vi "InitializeMaskLoad.vi"(4 "dxfFile":string, 5 "Masks":string, 6 "WaferTestPoints":string, 7 "DXFCanvas":refnum<k24>, 9 "TestPointsLoaded":bool, 10 "Wafer Definition File":path, 11 "MicrositesRef":refnum<k24>) -> (0 "error out":errorcluster, 3 "error out 5":errorcluster)   [LabVIEW 2020]
uses:
  C:/Users/User/Desktop/Automation/NextVersion/DXFViewer/LabviewDXFViewer/LabviewDXFViewer/bin/Release/LabviewDXFViewer.exe
  LabviewDXFViewer/bin/Release/LabviewDXFViewer.exe
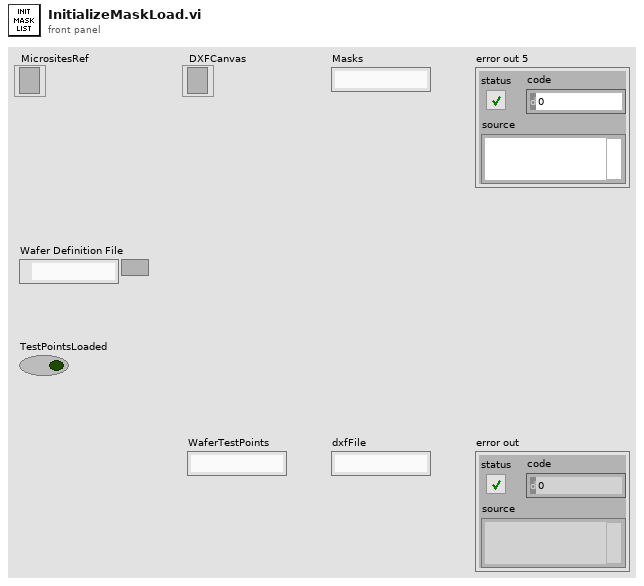
[diagram p1: front panel]
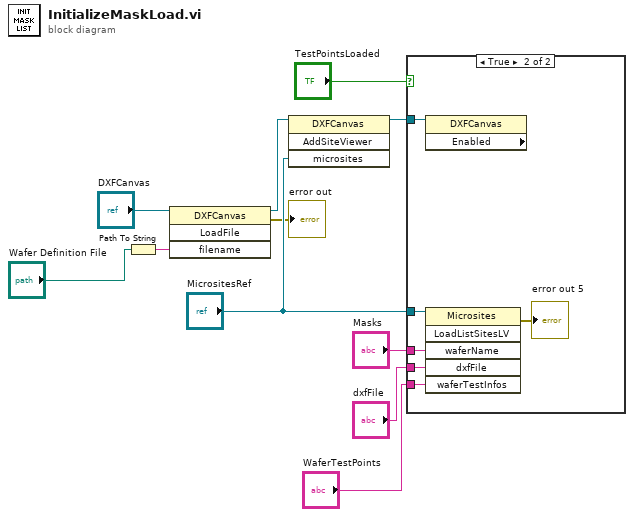
[diagram p0: block diagram]
diagram:
  n1 = Path To String(path="Wafer Definition File") -> (string=w3:string)
  n2 = invoke class="DXFCanvas" method="LoadFile"(reference="DXFCanvas", "filename"=w3) -> (reference out=w1:refnum<k24>, error out=→"error out":errorcluster)  [unwired: 2 in, 2 out]
  n3 = invoke class="DXFCanvas" method="AddSiteViewer"(reference=w1, "microsites"="MicrositesRef") -> (reference out=w9:refnum<k24>)  [unwired: 2 in, 3 out]
  n4 = case shown="True" "TestPointsLoaded" {
    tunnel: "Masks" -> [_ w17]
    tunnel: "MicrositesRef" -> [_ w16]
    tunnel: w9 -> [_ w14]
    tunnel: "WaferTestPoints" -> [_ w13]
    tunnel: "dxfFile" -> [_ w12]
    frame False {
    }
    frame True {
      n5 = property class="DXFCanvas" props=["Enabled"](reference=w14) -> ()  [unwired: 1 in, 3 out]
      n6 = invoke class="Microsites" method="LoadListSitesLV"(reference=w16, "waferName"=w17, "dxfFile"=w12, "waferTestInfos"=w13) -> (error out=→"error out 5":errorcluster)  [unwired: 2 in, 5 out]
    }
  }
